vi "SSH Unix Make Temp Pwd File.vi"(8 "error in (no error)":errorcluster, 11 "Password":string) -> (0 "error out":errorcluster, 3 "sshpass command prefix":string)   [LabVIEW 2019, in "LMH-LINX.lvlib"]
uses:
  <vilib>/MakerHub/LINX/LMH-LINX.lvlib
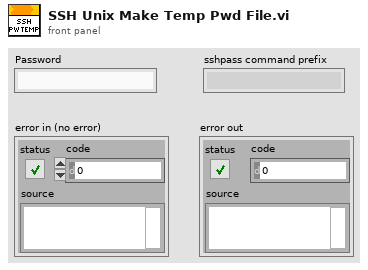
[diagram p1: front panel]
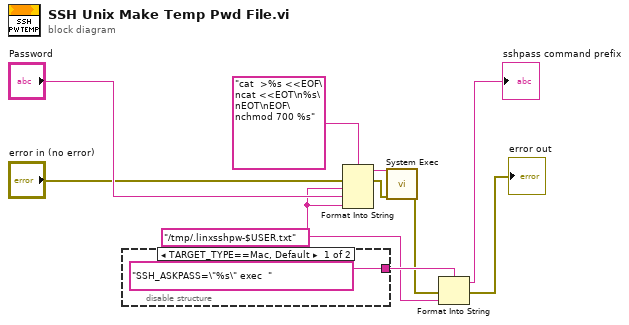
[diagram p0: block diagram]
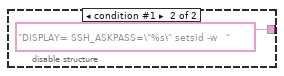
[diagram p2: hidden frame]
diagram:
  w5 = "/tmp/.linxsshpw-$USER.txt"
  n1 = disable-structure shown="TARGET_TYPE==Mac, Default" {
    disable-tunnel: ["SSH_ASKPASS=\"%s\" exec  " "DISPLAY= SSH_ASKPASS=\"%s\" setsid -w   "] -> w9
    frame condition #0 (active) {
    }
    frame condition #1 {
    }
  }
  n2 = Format Into String(format string="cat  >%s <<EOF\ncat <<EOT\n%s\nEOT\nEOF\nchmod 700 %s" ("command line"), error in="error in (no error)", w5, "Password", w5) -> (resulting string=w7:string, error out=w1:errorcluster)  [unwired: 1 in]
  n3 = call <vilib>:"System Exec.vi"("error in (no error)"=w1, "command line"=w7) -> ("error out"=w6:errorcluster)  [unwired: 6 in, 3 out]
  n4 = Format Into String(format string=w9, error in=w6, w5) -> (resulting string=→"sshpass command prefix":string, error out=→"error out":errorcluster)  [unwired: 1 in]
